vi "Write Single Holding Register.vi"(8 "error in":errorcluster, 9 "register to write":u16, 10 "address":u16, 11 "Modbus master in":refnum<class "Modbus Master.lvclass">) -> (0 "error out":errorcluster, 3 "Modbus master out":refnum<class "Modbus Master.lvclass">)   [LabVIEW 2014, in "MyLib.lvlib" / "Modbus Master.lvclass"]
doc: "Writes <B>register to write</B> to <B>address</B> of the device."
uses:
  Modbus Master.lvclass
  Modbus Master.lvclass/Modbus Master.ctl
  Modbus API.lvclass/Modbus API.ctl
  Transmission Data Unit/Transmission Data Unit.lvclass
  Master Function Definition/Master Function Definition.lvclass
  Modbus API.lvclass
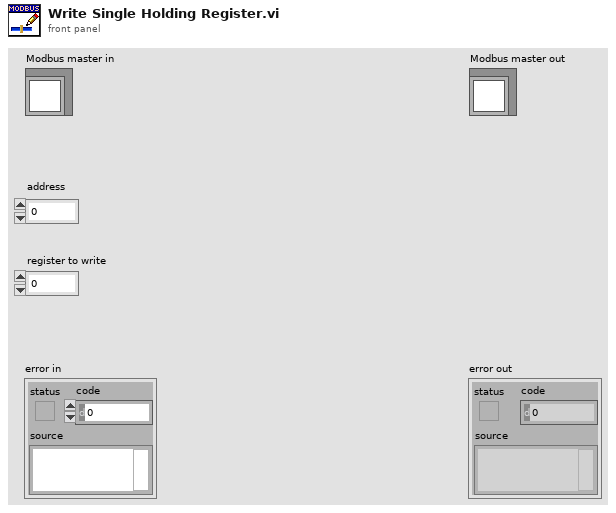
[diagram p1: front panel]
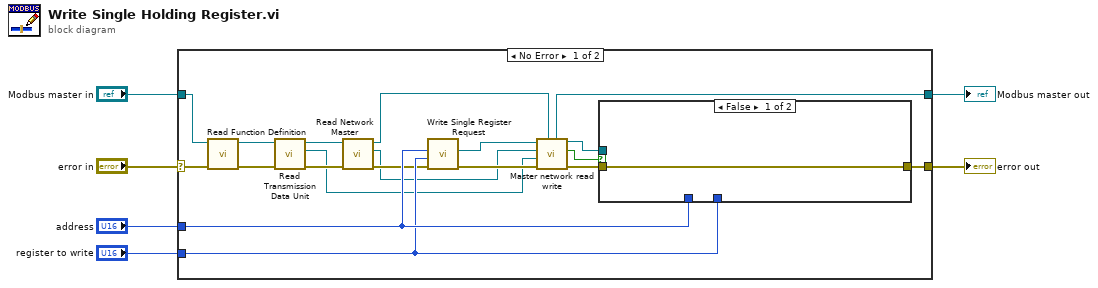
[diagram p0: block diagram]
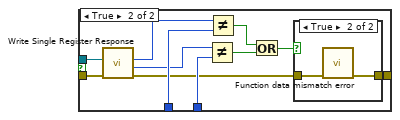
[diagram p2: hidden frame]
diagram:
  n1 = case shown="No Error" "error in" {
    selector: "error in" -> [w13 w41]
    tunnel: "Modbus master in" -> [w11 w42]
    tunnel: [w18 w42] -> w4
    tunnel: [w24 w41] -> w3
    tunnel: "address" -> [w23 _]
    tunnel: "register to write" -> [w22 _]
    frame No Error {
      n2 = call "Read Function Definition.vi"("error in"=w13, "Modbus master in"=w11) -> ("error out"=w16:errorcluster, "Modbus master out"=w15:refnum<class "Modbus Master.lvclass">)  [unwired: 7 in, 1 out]
      n3 = call "Read Transmission Data Unit.vi"("error in"=w16, "Modbus instance in"=w15) -> ("error out"=w14:errorcluster, "transmission data unit"=w9:refnum<class "Transmission Data Unit.lvclass">, "Modbus instance out"=w17:refnum<class "Modbus Master.lvclass">)  [unwired: 7 in]
      n4 = call "Read Network Master.vi"("error in"=w14, "Modbus master in"=w17) -> ("error out"=w12:errorcluster, "network master"=w8:refnum<class "Network Master.lvclass">, "Modbus master out"=w10:refnum<class "Modbus Master.lvclass">)  [unwired: 7 in]
      n5 = call "Write Single Register Request.vi"("error in"=w12, "Register Value"=w22, "Starting Address"=w23) -> ("error out"=w25:errorcluster, "modbus data unit out"=w20:refnum<class "Modbus Data Unit.lvclass">)  [unwired: 7 in]
      n6 = call "Master network read write.vi"("Modbus master in"=w10, "error in"=w25, "transmission data unit in"=w9, "network master in"=w8, "Modbus data unit in"=w20) -> ("error out"=w21:errorcluster, "PDU Valid?"=w7:bool, "Modbus data unit out"=w19:refnum<class "Modbus Data Unit.lvclass">, "Modbus master out"=w18:refnum<class "Modbus Master.lvclass">)  [unwired: 3 in]
      n7 = case shown="False" w7 {
        tunnel: [w26 w34] -> w24
        tunnel: w23 -> [_ w32]
        tunnel: w22 -> [_ w31]
        tunnel: w21 -> [w26 w29]
        tunnel: w19 -> [_ w28]
        frame False {
        }
        frame True {
          n8 = call "Write Single Register Response.vi"("error in"=w29, "modbus data unit in"=w28) -> ("error out"=w27:errorcluster, "Number of Coils"=w30:u16, "Address"=w33:u16)  [unwired: 7 in]
          n9 = Not Equal?(x=w30, y=w31) -> (x != y?=w37:bool)
          n10 = Not Equal?(x=w33, y=w32) -> (x != y?=w36:bool)
          n11 = Or(x=w36, y=w37) -> (x .or. y?=w35:bool)
          n12 = case shown="True" w35 {
            tunnel: [w38 w40] -> w34
            tunnel: w27 -> [w38 w39]
            frame False {
            }
            frame True {
              n13 = call "Function data mismatch error.vi"("error in (no error)"=w39) -> ("error out"=w40:errorcluster)  [unwired: 10 in]
            }
          }
        }
      }
    }
    frame Error {
    }
  }
  "error out" <- w3
  "Modbus master out" <- w4
